vi "PCAN_VERSION.vi"(8 "error in (no error)":errorcluster, 11 "path in":path) -> (0 "error out":errorcluster, 1 "path out":path, 2 "lpszTextBuff":string, 3 "error":T1 items=["CAN_ERR_OK"=0, "CAN_ERR_XMTFULL"=1, "CAN_ERR_OVERRUN"=2, "CAN_ERR_BUSLIGHT"=4, "CAN_ERR_BUSHEAVY"=8, "CAN_ERR_BUSOFF"=16, "CAN_ERR_QRCVEMPTY"=32, "CAN_ERR_QOVERRUN"=64, "CAN_ERR_QXMTFULL"=128, "CAN_ERR_REGTEST"=256, "CAN_ERR_NOVXD"=512, "CAN_ERR_HWINUSE"=1024, "CAN_ERR_NETINUSE"=2048, "CAN_ERR_ILLHW"=5120, "CAN_ERR_ILLNET"=6144, "CAN_ERR_ILLCLINET"=7168, "CAN_ERR_RESOURCE"=8192, "CAN_ERR_ILLPARAMTYPE"=16384, "CAN_ERR_ILLPARAMVAL"=32768, "CAN_ERR_UNKNOWN"=65536])   [LabVIEW 2017]
uses:
  CANalystII/PCAN_Driver/PCAN_ERROR.ctl
  CANalystII/PCAN_USB.dll
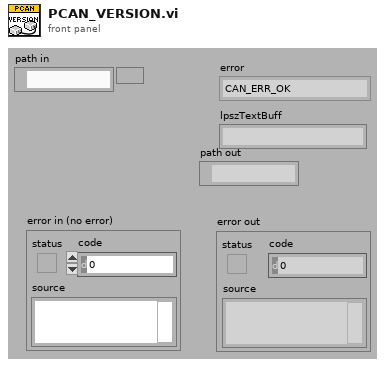
[diagram p1: front panel]
types:
  T1 = typedef "PCAN_ERROR.ctl" = i32
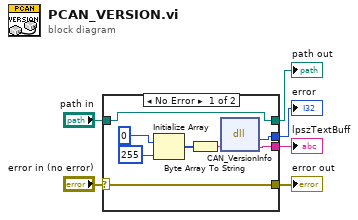
[diagram p0: block diagram]
diagram:
  n1 = case shown="No Error" "error in (no error)" {
    selector: "error in (no error)" -> [w13 w16]
    tunnel: [w14 _] -> w4
    tunnel: [w13 w16] -> w5
    tunnel: [w8 _] -> w3
    tunnel: "path in" -> [w7 w15]
    tunnel: [w7 w15] -> w1
    frame No Error {
      n2 = Initialize Array(u8 0 ("element"), 255 ("dimension size")) -> (w10:u8[])
      n3 = Byte Array To String(unsigned byte array=w10) -> (string=w9:string)
      n4 = dll-call lib="C:/Projects/Fuse_LW/Fuse25A_Labview/CANalystII/PCAN_USB.dll" fn="CAN_VersionInfo"("lpszTextBuff"=w9) -> ("return type"=w14:i32, "lpszTextBuff"=w8:string)  [unwired: 3 in, 2 out]
    }
    frame Error {
    }
  }
  "error out" <- w5
  "error" <- w4
  "lpszTextBuff" <- w3
  "path out" <- w1
